vi "FIRadaptiveQR1.vi"(5 "lambda":dbl=1.0, 7 "P1/2":dbl[][](array[numeric]), 10 "d":dbl, 11 "u":dbl) -> (3 "w":dbl[](array[numeric]))   [LabVIEW 2010, in "KevLib01.lvlib"]
uses:
  KevLib01.lvlib
  <vilib>/Analysis/Matrix/NI_Matrix.lvlib
  <vilib>/Analysis/NI_AALBase.lvlib
  <vilib>/Analysis/baseanly.llb/Vector x A.vi
  <vilib>/Analysis/NI_AALPro.lvlib
  <vilib>/Analysis/7linalg.llb/Real Transpose Matrix.vi
  <vilib>/Analysis/7linalg.llb/Real QR Decomposition.vi
  <vilib>/Analysis/baseanly.llb/Real Dot Product.vi
  <vilib>/Analysis/Matrix/Numeric/Conversions/Array To Matrix - RA2.vi
  <vilib>/Analysis/Matrix/Numeric/Multiply/Multiply - R,RM.vi
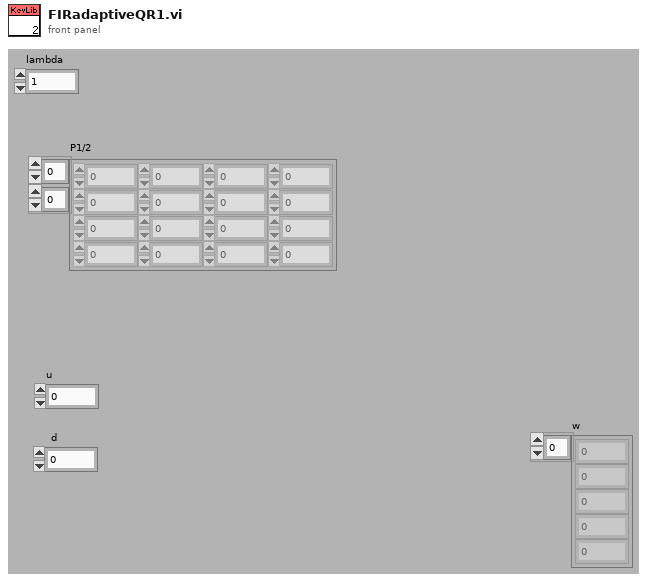
[diagram p1: front panel]
types:
  T1 = typedef "NI_Matrix.lvlib/RealMatrix.ctl" = dbl[][]
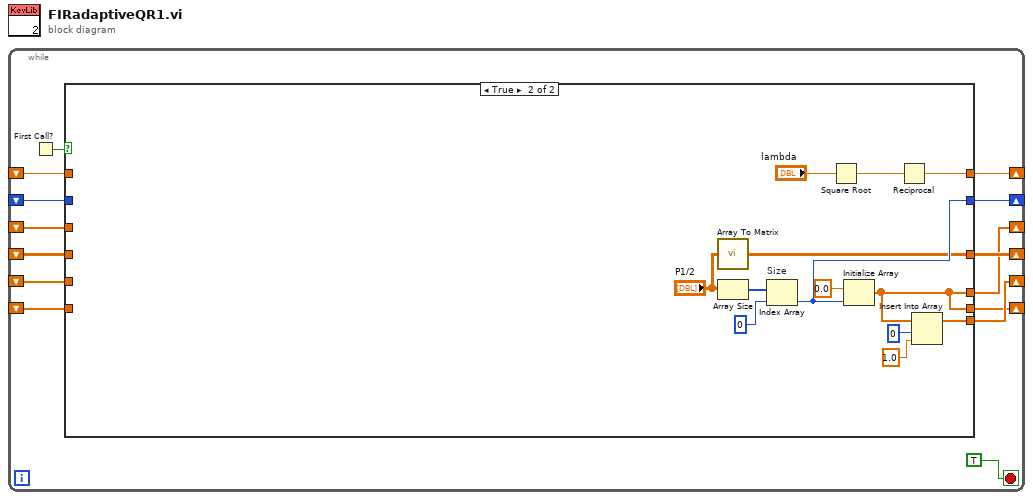
[diagram p0: block diagram]
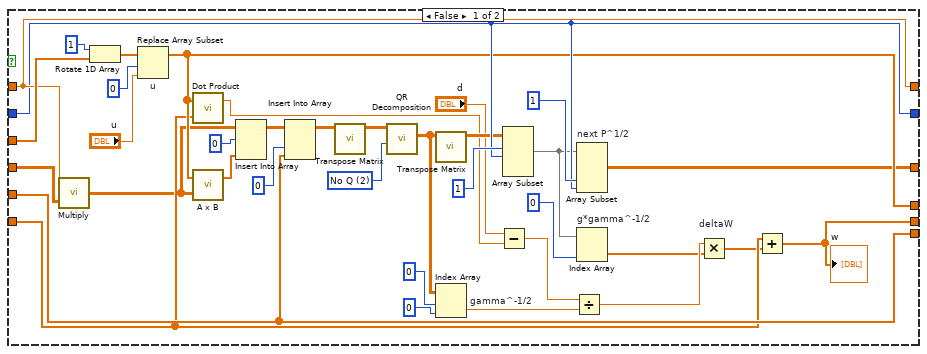
[diagram p2: hidden frame]
diagram:
  n1 = while {
    shift-right: [w13] -> _
    shift-left: _ -> [w12]
    shift-right: [w10] -> _
    shift-left: _ -> [w9]
    shift-right: [w8] -> _
    shift-left: _ -> [w5]
    shift-right: [w7] -> _
    shift-left: _ -> [w6]
    shift-right: [w4] -> _
    shift-left: _ -> [w3]
    shift-right: [w2] -> _
    shift-left: _ -> [w1]
    stop <- TRUE stop-if-true
    n2 = First Call?() -> (First Call?: T/F=w14:bool)
    n3 = case shown="True" w14 {
      tunnel: [w45 w57] -> w13
      tunnel: w12 -> [w45 _]
      tunnel: [w39 w60] -> w10
      tunnel: w9 -> [w39 _]
      tunnel: [w15 w51] -> w8
      tunnel: [w25 w53] -> w7
      tunnel: w6 -> [w50 _]
      tunnel: w5 -> [w27 _]
      tunnel: [w36 w54] -> w4
      tunnel: w3 -> [w36 _]
      tunnel: [w17 w53] -> w2
      tunnel: w1 -> [w23 _]
      frame False {
        w35 = u16 2 items=["Full Size Q", "Economy Size Q", "No Q"] ("Q option")
        n4 = call-poly <vilib>:"Multiply.vi"("Real Matrix A"=w27, "Real Scalar c"=w45) -> ("c * A"=w16:T1)
        n5 = Rotate 1D Array(1:w50, 2:1 ("n")) -> (0:w48:dbl[])
        n6 = Replace Array Subset "u"(array=w48, new element="u", index=0) -> (w25:dbl[])
        n7 = call-poly <vilib>:"Dot Product.vi"("Y Vector"=w23, "X Vector"=w25) -> ("X * Y"=w24:dbl)  [unwired: 1 out]
        n8 = call-poly <vilib>:"A x B.vi"("Matrix A"=w16, "Vector V'"=w25) -> ("V' x A"=w44:dbl[])  [unwired: 1 out]
        n9 = Insert Into Array(array=w16, index (row)=0, new element=w44) -> (w34:T1)  [unwired: 1 in]
        n10 = Insert Into Array(array=w34, index (col)=0 ("disabled index (col)"), new element=w36) -> (w33:T1)  [unwired: 1 in]
        n11 = call-poly <vilib>:"Transpose Matrix.vi"("Input Matrix"=w33) -> ("Matrix Transpose"=w32:T1)  [unwired: 10 out]
        n12 = call-poly <vilib>:"QR Decomposition.vi"("Q option"=w35, "A"=w32) -> ("R"=w30:T1)  [unwired: 1 in, 8 out]
        n13 = call-poly <vilib>:"Transpose Matrix.vi"("Input Matrix"=w30) -> ("Matrix Transpose"=w31:T1)  [unwired: 10 out]
        n14 = Index Array "gamma^-1/2"(array=w30, index (row)=0, index (col)=0 ("disabled index (col)")) -> (element=w21:dbl)
        n15 = Subtract(x="d", y=w24) -> (x-y=w22:dbl)
        n16 = Array Subset(array=w31, index (row)=1 ("index"), length (row)=w39) -> (w38:T1)  [unwired: 2 in]
        n17 = Divide(x=w22, y=w21) -> (x/y=w20:dbl)
        n18 = Array Subset "next P^1/2"(array=w38, index (col)=1 ("index"), length (col)=w39) -> (w15:T1)  [unwired: 2 in]
        n19 = Index Array "g*gamma^-1/2"(array=w38, index (col)=0 ("disabled index (col)")) -> (element=w19:dbl[])  [unwired: 1 in]
        n20 = Multiply "deltaW"(x=w20, y=w19) -> (x*y=w18:dbl[])
        n21 = Add(x=w23, y=w18) -> (x+y=w17:dbl[])
        "w" <- w17
      }
      frame True {
        n22 = call-poly <vilib>:"Array To Matrix.vi"("Real 2D Array"="P1/2") -> ("Real Matrix"=w51:T1)
        n23 = Array Size(array="P1/2") -> (size(s)=w63:i32[])
        n24 = Index Array "Size"(array=w63, index=0) -> (element=w60:i32)
        n25 = Square Root(x="lambda") -> (sqrt(x)=w59:dbl)
        n26 = Initialize Array(0.0 ("element"), w60) -> (w53:dbl[])
        n27 = Reciprocal(x=w59) -> (1/x=w57:dbl)
        n28 = Insert Into Array(array=w53, index=0, new element=1.0 ("new element/subarray")) -> (w54:dbl[])
      }
    }
  }
